vi "Read Displacements in Summary.vi"(11 "StiffnessCalculator in":refnum<class "StiffnessCalculator.lvclass">) -> (2 "Displacements in Summary":dbl[unit][](array[numeric]) min=-0.19963032420594115 max=0.19963032420594115 format="%.2f", 3 "StiffnessCalculator out":refnum<class "StiffnessCalculator.lvclass">)   [LabVIEW 2015, in "StiffnessCalculator.lvclass"]
uses:
  StiffnessCalculator.lvclass
  StiffnessCalculator.lvclass/StiffnessCalculator.ctl
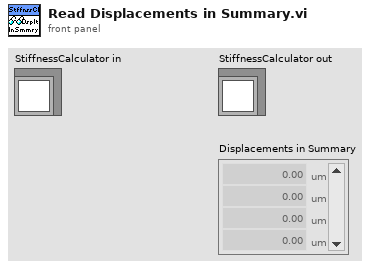
[diagram p1: front panel]
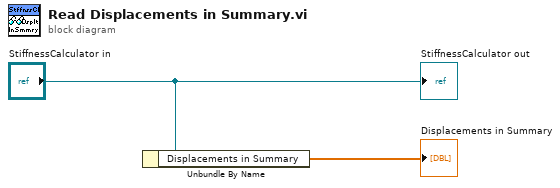
[diagram p0: block diagram]
diagram:
  n1 = Unbundle By Name("StiffnessCalculator in") -> ("Displacements in Summary"=→"Displacements in Summary":dbl[unit][])
  "StiffnessCalculator out" <- "StiffnessCalculator in"
